vi "ArmNetwork.vi"(8 "error in (no error)":errorcluster) -> (0 "error out":errorcluster)   [LabVIEW 2023]
doc: "Network for Arm\n\nInputs:\n -- error in -- cluster\n\nOutputs:\n -- error in -- cluster"
uses:
  <vilib>/Rock Robotics/Network Tables/NT Write Boolean.vi
  <vilib>/Rock Robotics/Network Tables/NT Write Number.vi
  ArmGlobal.vi
  <vilib>/Rock Robotics/Network Tables/NT Write String.vi
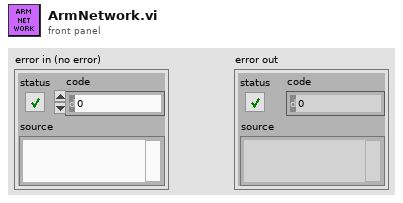
[diagram p1: front panel]
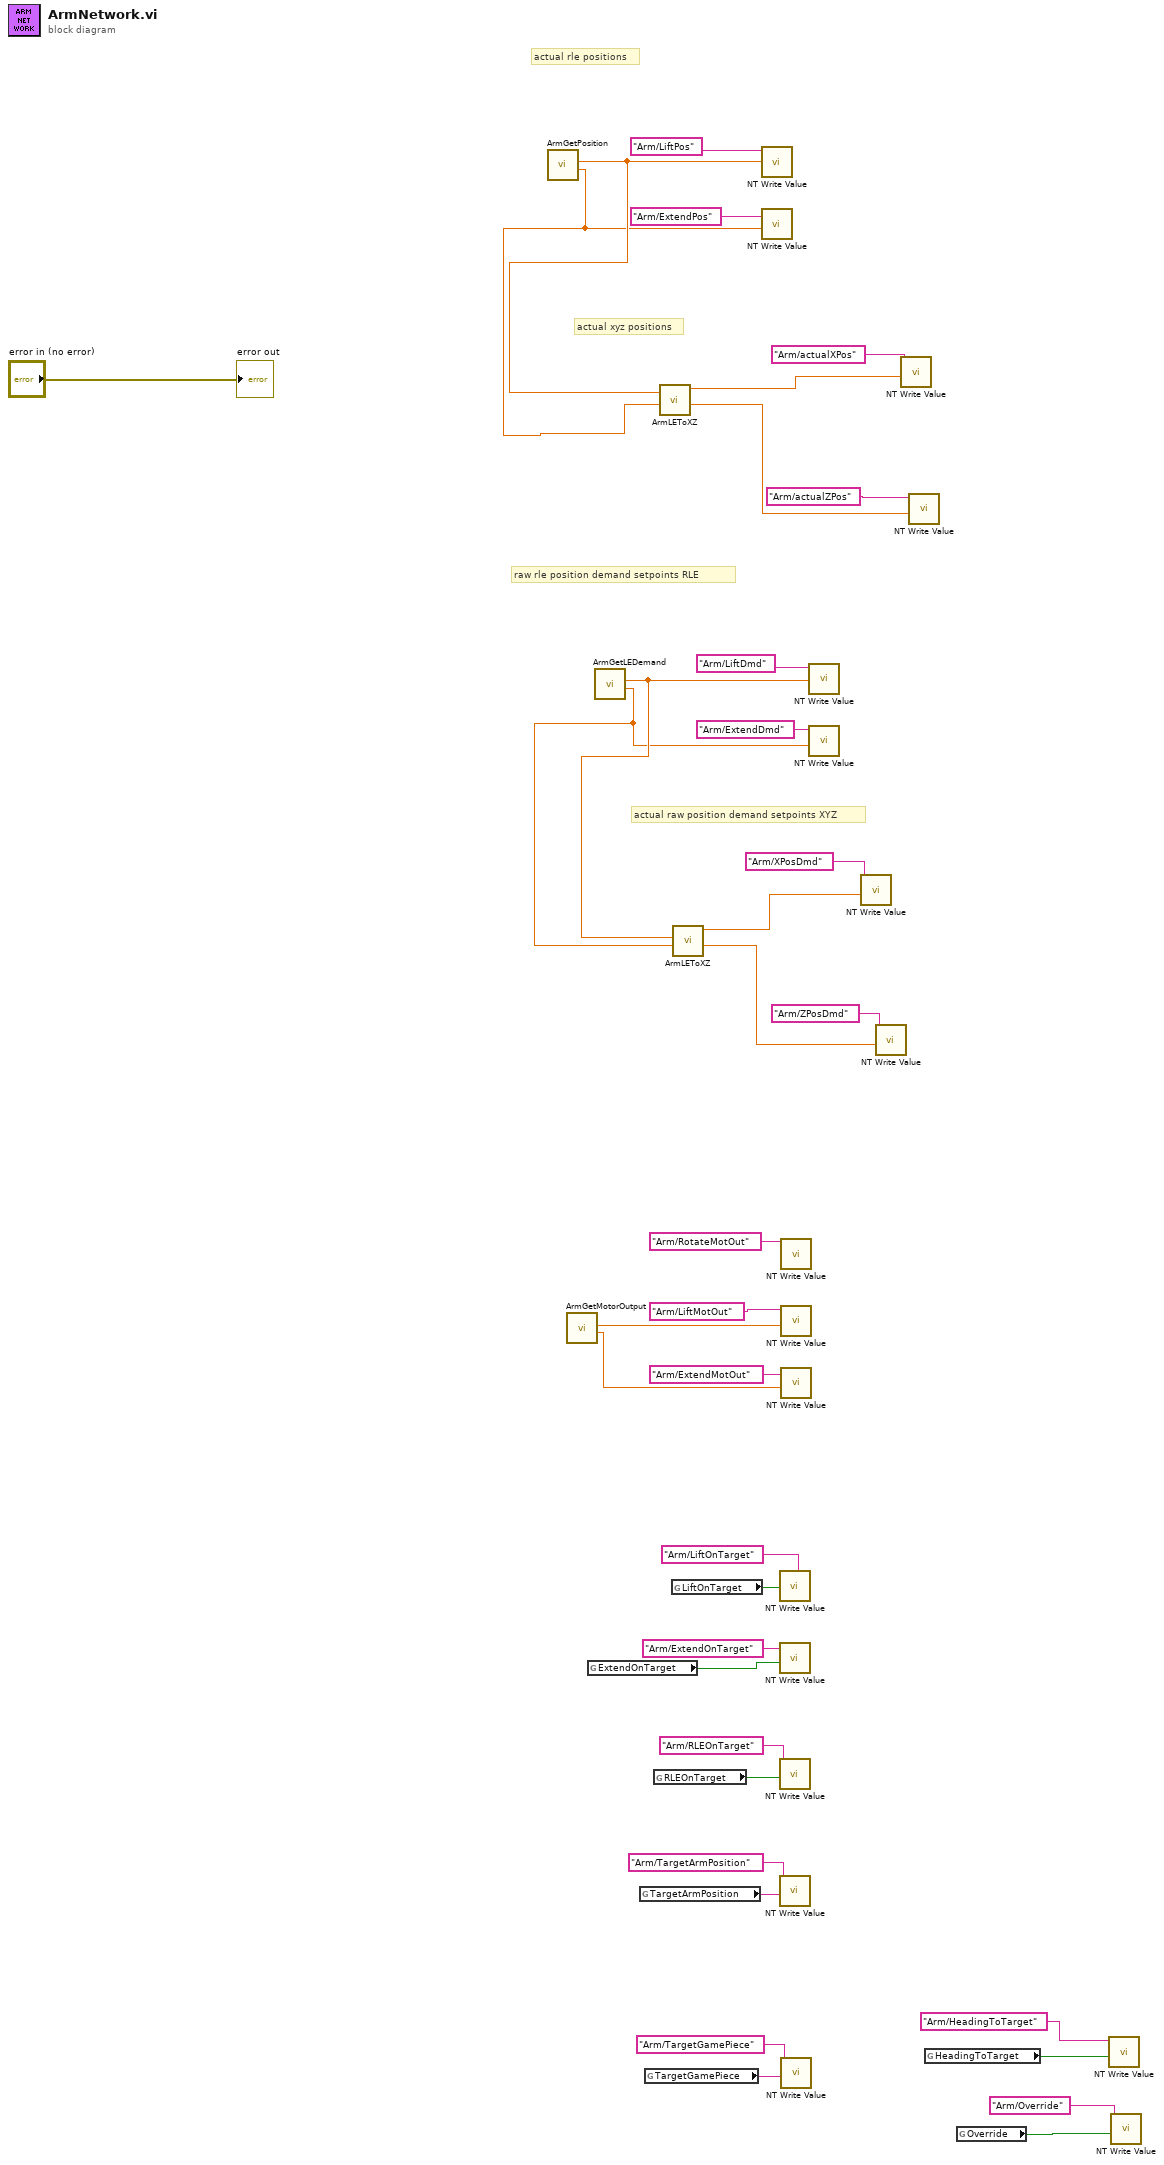
[diagram p0: block diagram]
diagram:
  # "actual xyz positions"
  # "actual raw position demand setpoints XYZ"
  # "actual rle positions"
  # "raw rle position demand setpoints RLE"
  n1 = call "ArmGetPosition.vi"() -> ("ExtendPostion"=w11:dbl, "LiftPostion"=w16:dbl)  [unwired: 10 in]
  n2 = call "ArmGetMotorOutput.vi"() -> ("ExtendMotorOutput"=w34:dbl, "LiftMotorOutput"=w35:dbl)  [unwired: 10 in]
  n3 = global read "ArmGlobal.vi" "ExtendOnTarget"() -> (w24:bool)
  n4 = call "ArmGetLEDemand.vi"() -> ("ExtendPositonDemand(in)"=w9:dbl, "LiftPositionDemand(d)"=w10:dbl)  [unwired: 10 in]
  n5 = global read "ArmGlobal.vi" "TargetArmPosition"() -> (w20:string)
  n6 = global read "ArmGlobal.vi" "TargetGamePiece"() -> (w18:string)
  n7 = global read "ArmGlobal.vi" "RLEOnTarget"() -> (w22:bool)
  n8 = call "ArmLEToXZ.vi"("Extend"=w11, "Lift"=w16) -> ("z"=w14:dbl, "x"=w15:dbl)  [unwired: 8 in]
  n9 = global read "ArmGlobal.vi" "LiftOnTarget"() -> (w26:bool)
  n10 = call "ArmLEToXZ.vi"("Extend"=w9, "Lift"=w10) -> ("z"=w7:dbl, "x"=w8:dbl)  [unwired: 8 in]
  n11 = call-poly <vilib>:"NT Write Value.vi"("value"=w16, "name"="Arm/LiftPos") -> ()  [unwired: 9 in, 1 out]
  n12 = call-poly <vilib>:"NT Write Value.vi"("value"=w11, "name"="Arm/ExtendPos") -> ()  [unwired: 9 in, 1 out]
  n13 = call-poly <vilib>:"NT Write Value.vi"("value"=w26, "name"="Arm/LiftOnTarget") -> ()  [unwired: 9 in, 1 out]
  n14 = call-poly <vilib>:"NT Write Value.vi"("value"=w24, "name"="Arm/ExtendOnTarget") -> ()  [unwired: 9 in, 1 out]
  n15 = call-poly <vilib>:"NT Write Value.vi"("value"=w22, "name"="Arm/RLEOnTarget") -> ()  [unwired: 9 in, 1 out]
  n16 = call-poly <vilib>:"NT Write Value.vi"("value"=w20, "name"="Arm/TargetArmPosition") -> ()  [unwired: 9 in, 1 out]
  n17 = call-poly <vilib>:"NT Write Value.vi"("name"="Arm/RotateMotOut") -> ()  [unwired: 10 in, 1 out]
  n18 = call-poly <vilib>:"NT Write Value.vi"("value"=w35, "name"="Arm/LiftMotOut") -> ()  [unwired: 9 in, 1 out]
  n19 = call-poly <vilib>:"NT Write Value.vi"("value"=w34, "name"="Arm/ExtendMotOut") -> ()  [unwired: 9 in, 1 out]
  n20 = call-poly <vilib>:"NT Write Value.vi"("value"=w18, "name"="Arm/TargetGamePiece") -> ()  [unwired: 9 in, 1 out]
  n21 = call-poly <vilib>:"NT Write Value.vi"("value"=w10, "name"="Arm/LiftDmd") -> ()  [unwired: 9 in, 1 out]
  n22 = call-poly <vilib>:"NT Write Value.vi"("value"=w9, "name"="Arm/ExtendDmd") -> ()  [unwired: 9 in, 1 out]
  n23 = call-poly <vilib>:"NT Write Value.vi"("value"=w8, "name"="Arm/XPosDmd") -> ()  [unwired: 9 in, 1 out]
  n24 = call-poly <vilib>:"NT Write Value.vi"("value"=w7, "name"="Arm/ZPosDmd") -> ()  [unwired: 9 in, 1 out]
  n25 = call-poly <vilib>:"NT Write Value.vi"("value"=w15, "name"="Arm/actualXPos") -> ()  [unwired: 9 in, 1 out]
  n26 = call-poly <vilib>:"NT Write Value.vi"("value"=w14, "name"="Arm/actualZPos") -> ()  [unwired: 9 in, 1 out]
  n27 = global read "ArmGlobal.vi" "HeadingToTarget"() -> (w4:bool)
  n28 = global read "ArmGlobal.vi" "Override"() -> (w2:bool)
  n29 = call-poly <vilib>:"NT Write Value.vi"("value"=w4, "name"="Arm/HeadingToTarget") -> ()  [unwired: 9 in, 1 out]
  n30 = call-poly <vilib>:"NT Write Value.vi"("value"=w2, "name"="Arm/Override") -> ()  [unwired: 9 in, 1 out]
  "error out" <- "error in (no error)"
